vi "SPCConfiguration.vi"(1 "Set/Get":bool, 2 "SPC Configuration (input)":T1={"SPC Initialization File"=path "SPC Labview Drivers/Important/spcm.ini", "Module Number"=0, "Operation Mode"=0, "Trigger Channel"="0"}) -> (0 "SPC Configuration (output)":T1={"SPC Initialization File"=path "SPC Labview Drivers/Important/spcm.ini", "Module Number"=0, "Operation Mode"=0, "Trigger Channel"="0"})   [LabVIEW 2009]
uses:
  SPCConfiguration.ctt
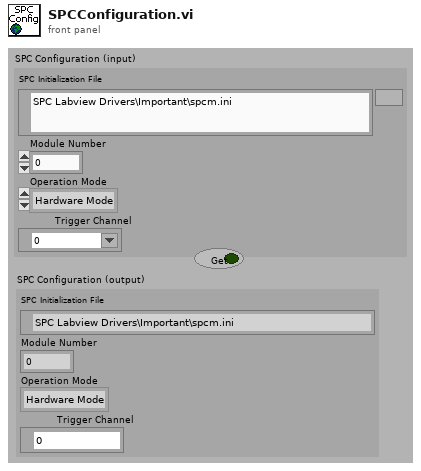
[diagram p1: front panel]
types:
  T1 = typedef "SPCConfiguration.ctt" = cluster{"SPC Initialization File":path, "Module Number":u16, "Operation Mode":u16, "Trigger Channel":tag}
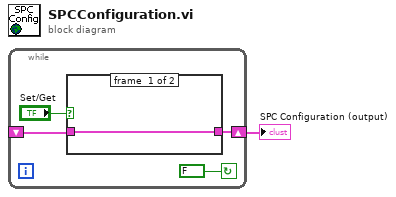
[diagram p0: block diagram]
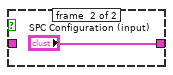
[diagram p2: hidden frame]
diagram:
  n1 = while {
    shift-right: [w4] -> w1
    shift-left: _ -> [w3]
    stop <- FALSE continue-if-true
    n2 = case shown="True" "Set/Get" {
      tunnel: [w6 "SPC Configuration (input)"] -> w4
      tunnel: w3 -> [w6 _]
      frame #0 {
      }
      frame #1 {
      }
    }
  }
  "SPC Configuration (output)" <- w1
